vi "SubVI_ReadTDMsAll.vi"(8 "error in":errorcluster, 10 "Range Slide":cluster{dbl, dbl}={0.0, 1.0}, 11 "tdms文件输出":refnum<k34>) -> (0 "error out":errorcluster, 1 "wfm name":string[](array[string]), 2 "WFM Out":waveform(dbl)[](array[waveform]), 3 "tdms file out":refnum<k34>, 4 "wfm Info":T1(array[cluster]))   [LabVIEW 2012]
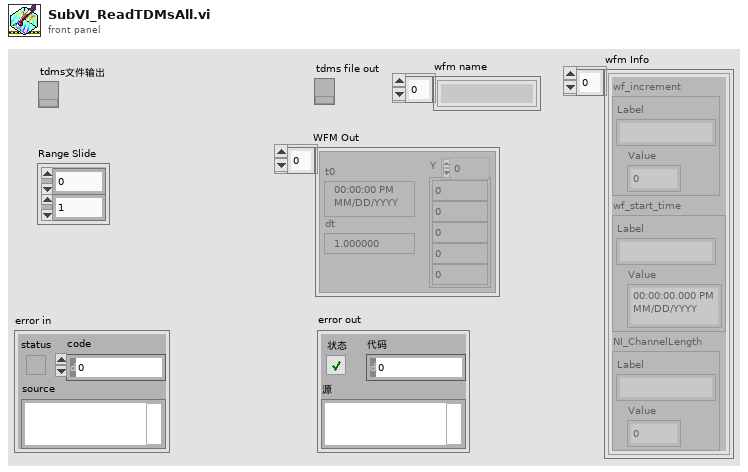
[diagram p1: front panel]
types:
  T1 = cluster{"wf_increment":cluster{"Label":string, "Value":dbl}, "wf_start_time":cluster{"Label":string, "Value":timestamp}, "NI_ChannelLength":cluster{"Label":string, "Value":dbl}}[]
  T2 = cluster{"wf_increment":cluster{"Label":string, "Value":dbl}, "wf_start_time":cluster{"Label":string, "Value":timestamp}, "NI_ChannelLength":cluster{"Label":string, "Value":dbl}}
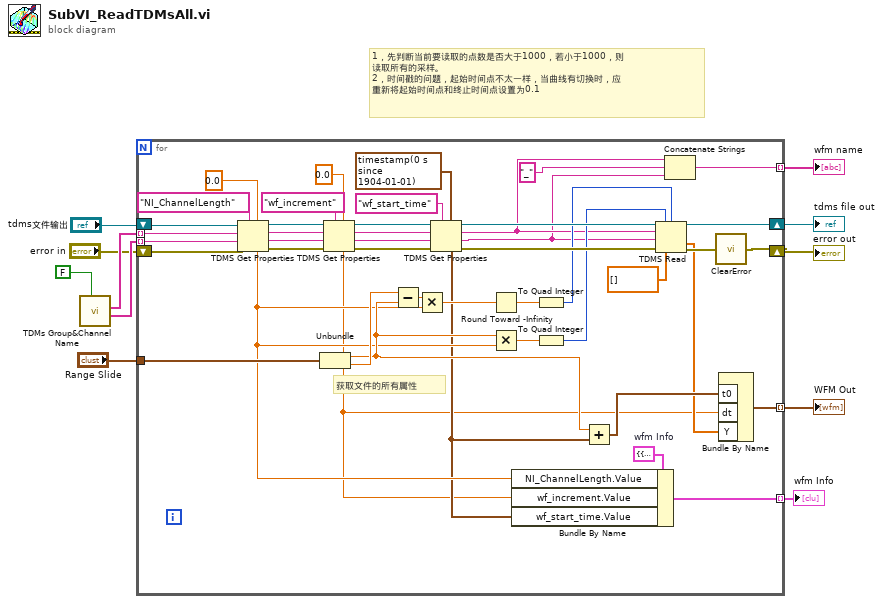
[diagram p0: block diagram]
diagram:
  # "1，先判断当前要读取的点数是否大于1000，若小于1000，则\n读取所有的采样。\n2，时间戳的问题，起始时间点不太一样，当曲线有切换时，应\n重新将起始时间点和终止时间点设置为0.1"
  n1 = call "TDMs Group&Channel Name.vi"("Ini?"=FALSE) -> ("Channel"=w9:string[], "Group"=w10:string[])  [unwired: 8 in, 1 out]
  n2 = for {
    tunnel: [w56] -> w6 mode=indexing
    tunnel: w10 -> [w53] mode=indexing
    tunnel: w9 -> [w33] mode=indexing
    shift-right: [w31] -> w8
    shift-left: "tdms文件输出" -> [w55]
    shift-right: [w32] -> w7
    shift-left: "error in" -> [w54]
    tunnel: "Range Slide" -> [w30]
    tunnel: [w17] -> w2 mode=indexing
    tunnel: [w13] -> w1 mode=indexing
    w16 = T2 {"wf_increment"={"Label"="wf_increment", "Value"=0.0}, "wf_start_time"={"Label"="wf_start_time", "Value"=timestamp(0 s since 1904-01-01)}, "NI_ChannelLength"={"Label"="NI_ChannelLength", "Value"=0.0}}  # wfm Info
    # "获取文件的所有属性"
    n3 = TDMS Get Properties(5:0.0, 7:"NI_ChannelLength", 8:w54, 9:w33, 10:w53, 11:w55) -> (0:w43:errorcluster, 1:w44:string, 2:w45:string, 3:w46:refnum<k34>, 4:w15:dbl)  [unwired: 1 out]
    n4 = Unbundle(w30) -> (w29:dbl, w50:dbl)
    n5 = TDMS Get Properties(5:0.0, 7:"wf_increment", 8:w43, 9:w44, 10:w45, 11:w46) -> (0:w39:errorcluster, 1:w35:string, 2:w37:string, 3:w41:refnum<k34>, 4:w12:dbl)  [unwired: 1 out]
    n6 = Subtract(x=w50, y=w29) -> (x-y=w34:dbl)
    n7 = Multiply(x=w34, y=w15) -> (x*y=w24:dbl)
    n8 = TDMS Get Properties(5:timestamp(0 s since 1904-01-01), 7:"wf_start_time" ("属性名称"), 8:w39, 9:w35, 10:w37, 11:w41) -> (0:w38:errorcluster, 1:w18:string, 2:w20:string, 3:w40:refnum<k34>, 4:w14:timestamp)  [unwired: 1 out]
    n9 = Round Toward -Infinity(1:w24) -> (0:w28:dbl)
    n10 = Multiply(x=w29, y=w15) -> (x*y=w49:dbl)
    n11 = Bundle By Name(cluster=w16, "NI_ChannelLength.Value"=w15, "wf_increment.Value"=w12, "wf_start_time.Value"=w14) -> (w13:T2)
    n12 = To Quad Integer(1:w28) -> (0:w23:i64)
    n13 = To Quad Integer(1:w49) -> (0:w21:i64)
    n14 = Add(x=w29, y=w14) -> (x+y=w26:timestamp)
    n15 = TDMS Read(0:w40, 1:w21, 2:w23, 5:w20, 7:w18, 11:w38, 12:dbl[] []) -> (4:w31:refnum<k34>, 10:w22:dbl[], 15:w25:errorcluster)  [unwired: 1 in, 3 out]
    n16 = Concatenate Strings(w20, "_" ("字符串"), w18) -> (w17:string)
    n17 = call <vilib>:"ClearError.vi"("error in (no error)"=w25) -> ("error out"=w32:errorcluster)
    n18 = Bundle By Name("t0"=w26, "dt"=w12, "Y"=w22) -> (w56:waveform(dbl))  [unwired: 1 in]
  }
  "tdms file out" <- w8
  "error out" <- w7
  "WFM Out" <- w6
  "wfm name" <- w2
  "wfm Info" <- w1
